vi "DOE Drying Rate Calculation.vi"(8 "Error In":errorcluster, 9 "RMC Data":dbl[](array[numeric]), 10 "Time (sec)":dbl[](array[numeric]), 11 "Slope Data In":dbl[](array[numeric])) -> (0 "Error Out":errorcluster, 2 "Drying Rate (%/min)":dbl, 3 "Slope Data Out":dbl[](array[numeric]))   [LabVIEW 2016]
uses:
  <vilib>/Analysis/NI_AALPro.lvlib
panel:
  out "XY Graph":cluster{"Y":dbl[], "Y":dbl[]}[](graph)
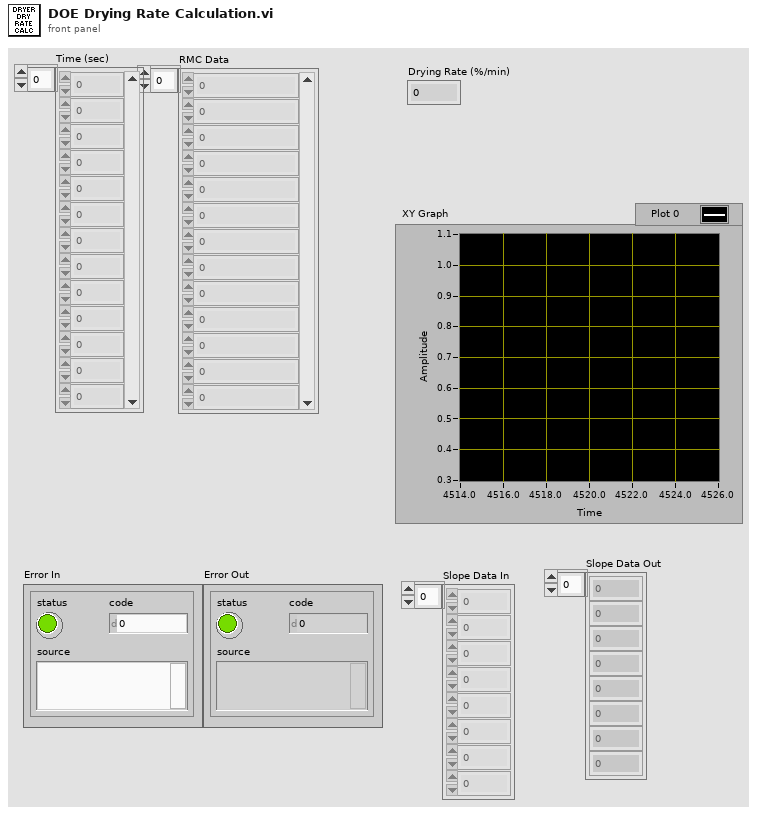
[diagram p1: front panel]
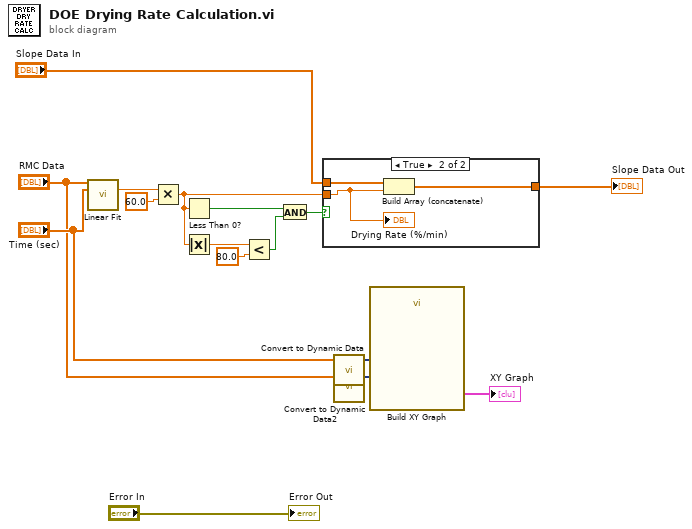
[diagram p0: block diagram]
diagram:
  n1 = call <vilib>:"Linear Fit.vi"("Y"="RMC Data", "X"="Time (sec)") -> ("slope"=w9:dbl)  [unwired: 9 in, 4 out]
  n2 = Multiply(x=w9, y=60.0) -> (x*y=w1:dbl)
  n3 = Less Than 0?(x=w1) -> (x < 0?=w12:bool)
  n4 = Absolute Value(x=w1) -> (abs(x)=w13:dbl)
  n5 = Less?(x=w13, y=80.0) -> (x < y?=w15:bool)
  n6 = And(x=w12, y=w15) -> (x .and. y?=w16:bool)
  n7 = case shown="True" w16 {
    tunnel: w1 -> [_ w18]
    tunnel: "Slope Data In" -> [w17 w20]
    tunnel: [w17 w19] -> w11
    frame False {
    }
    frame True {
      n8 = Build Array (concatenate)(w20, w18) -> (w19:dbl[])
      "Drying Rate (%/min)" <- w18
    }
  }
  "Slope Data Out" <- w11
  n9 = call "Convert to Dynamic Data"("Array"="Time (sec)") -> ("Dynamic Data Type"=w4:dynamicdata)  [unwired: 3 in]
  n10 = call "Convert to Dynamic Data2"("Array"="RMC Data") -> ("Dynamic Data Type"=w2:dynamicdata)  [unwired: 3 in]
  n11 = call "Build XY Graph"("Y Input"=w2, "X Input"=w4) -> ("XY Graph"=→"XY Graph":cluster{"X":dbl[], "Y":dbl[]}[])  [unwired: 8 in, 1 out]
  "Error Out" <- "Error In"
